vi "Control_NextPlayer.vi"(2 "Player":u8) -> (16 "NextPlayer":u8)   [LabVIEW 2018]
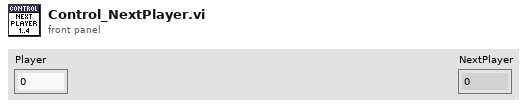
[diagram p1: front panel]
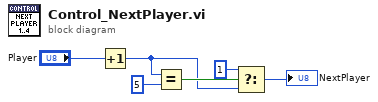
[diagram p0: block diagram]
diagram:
  n1 = Increment(x="Player") -> (x+1=w4:u8)
  n2 = Equal?(x=w4, y=u8 5) -> (x = y?=w6:bool)
  n3 = Select(t=u8 1, s=w6, f=w4) -> (s? t:f=→"NextPlayer":u8)
